vi "Source Live Profile.vi"(9 "Source Profile File":path, 10 "Simulate/Run":T1=enum."Run VI") -> (0 "error IO":errorcluster, 1 "Source Profile Out":path)   [LabVIEW 2021]
uses:
  Anemometry/Anemometry Sub Vis/Controls/User_Specific_mode.ctl
  Anemometry/Anemometry Sub Vis/Globals/Trav_pos_global.vi
  Anemometry/Anemometry Sub Vis/Globals/Meas_global.vi
panel:
  out "Initial Trace Voltage":dbl
  out "Initial Source Strength":dbl
  out "Control Trace Gas":bool
  out "Source Value":dbl format="%.2f"
  out "Time (s)":dbl[](array[numeric])
  out "XY Graph":cluster{dbl[], dbl[]}(graph)
  out "Source State":dbl[](array[numeric])
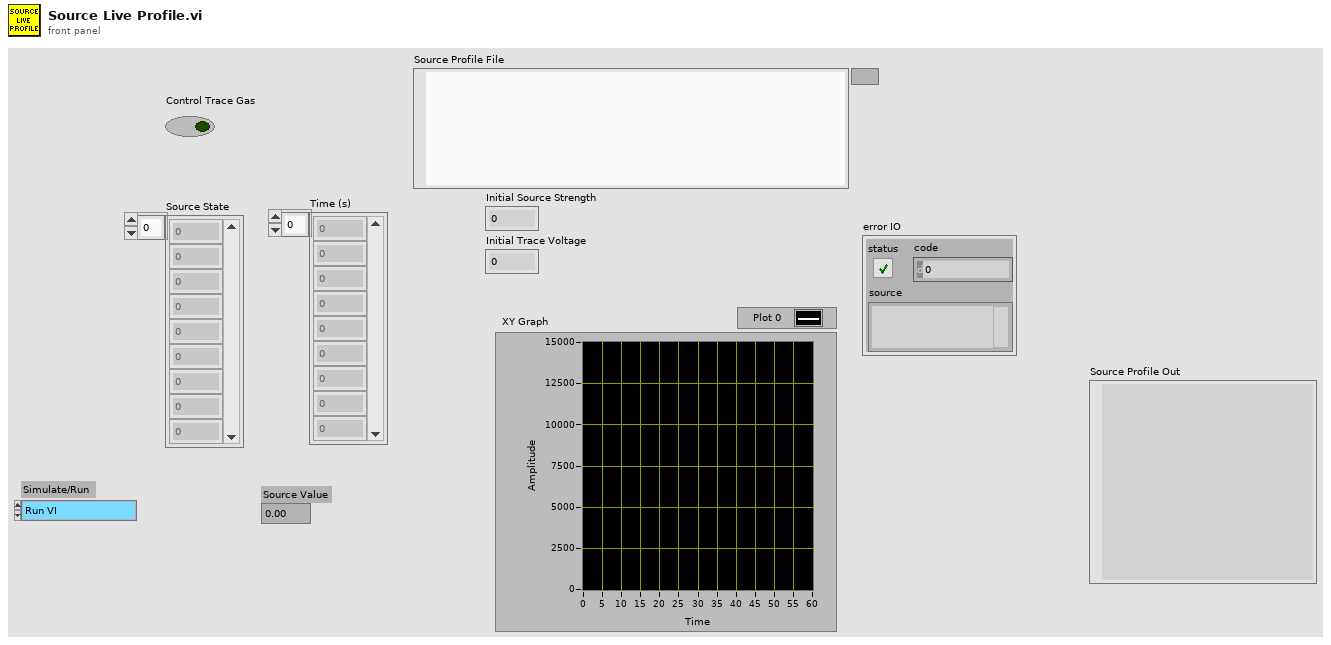
[diagram p1: front panel]
types:
  T1 = typedef "User_Specific_mode.ctl" = enum16{"Check VI only", "Run VI"}
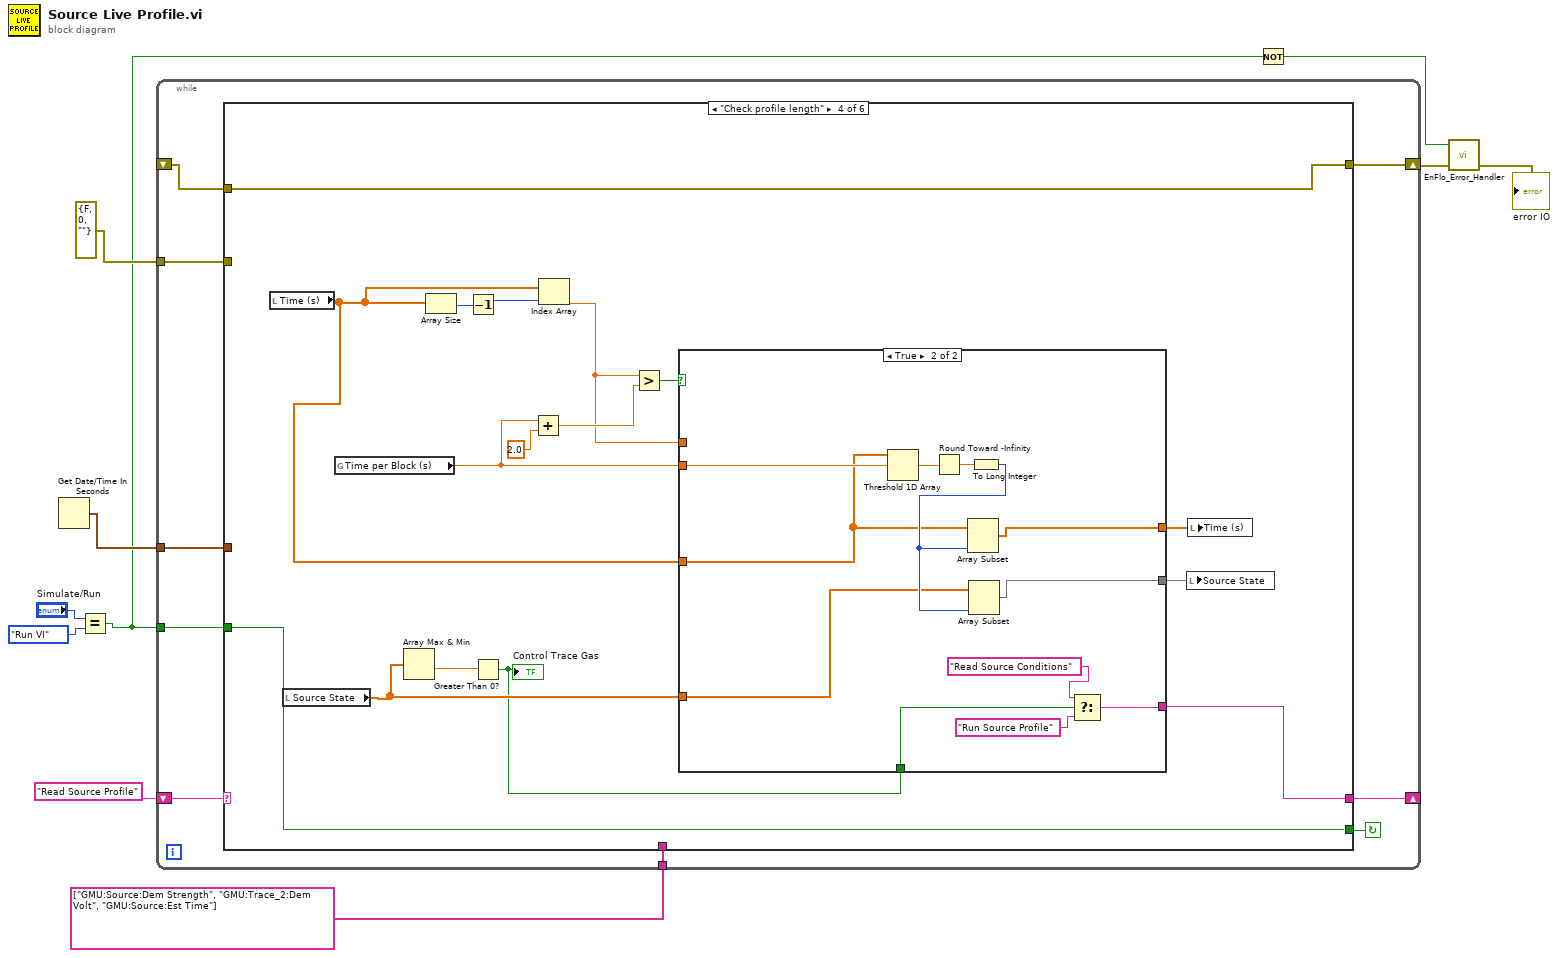
[diagram p0: block diagram]
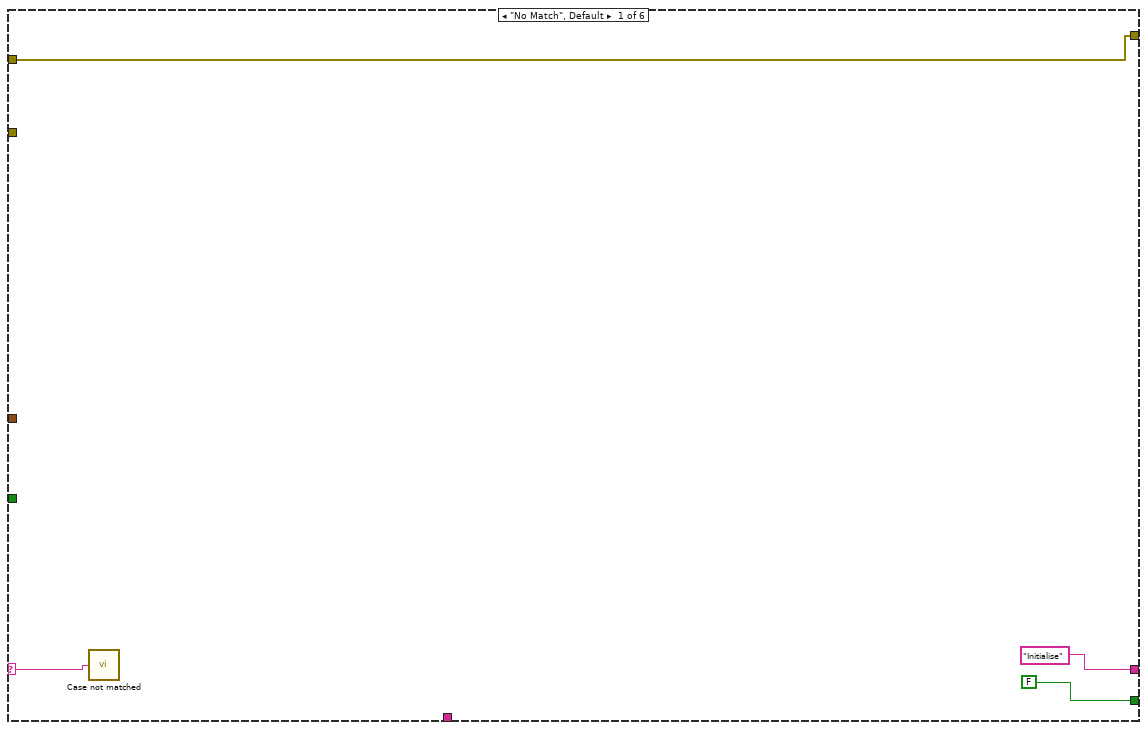
[diagram p2: hidden frame]
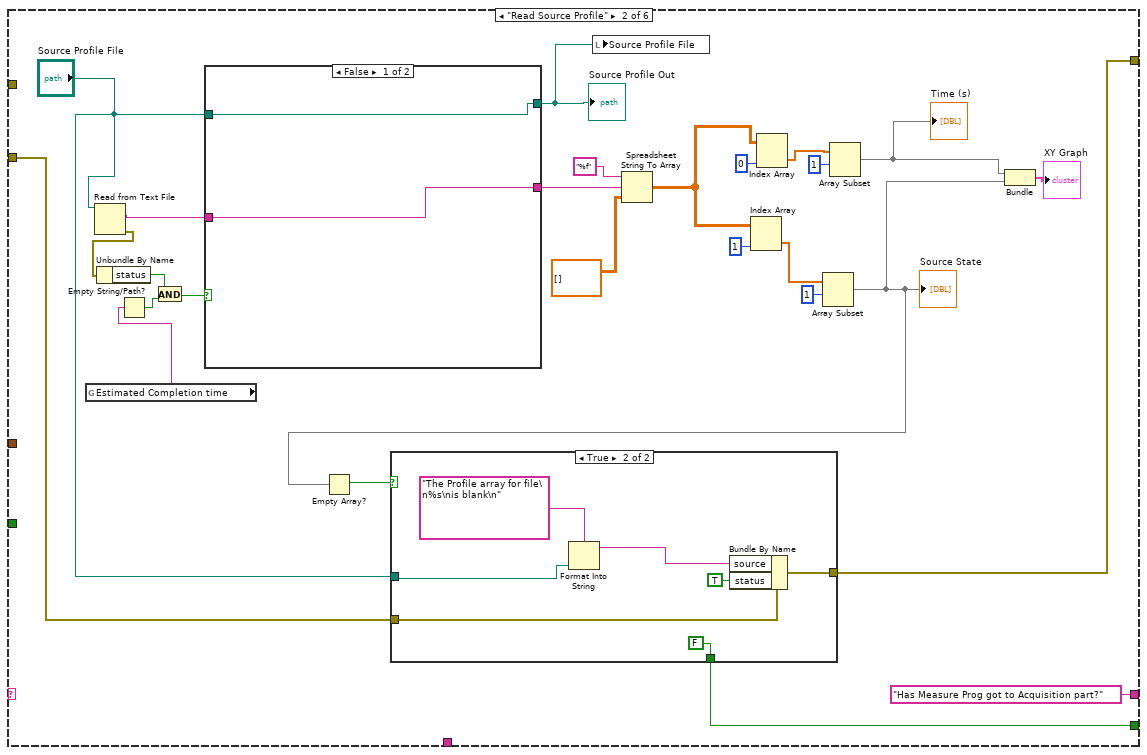
[diagram p3: hidden frame]
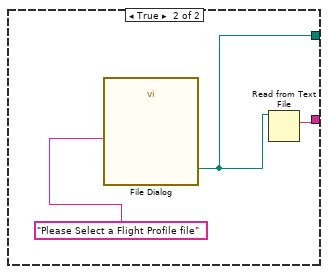
[diagram p4: hidden frame]
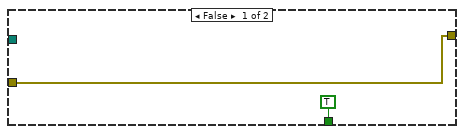
[diagram p5: hidden frame]
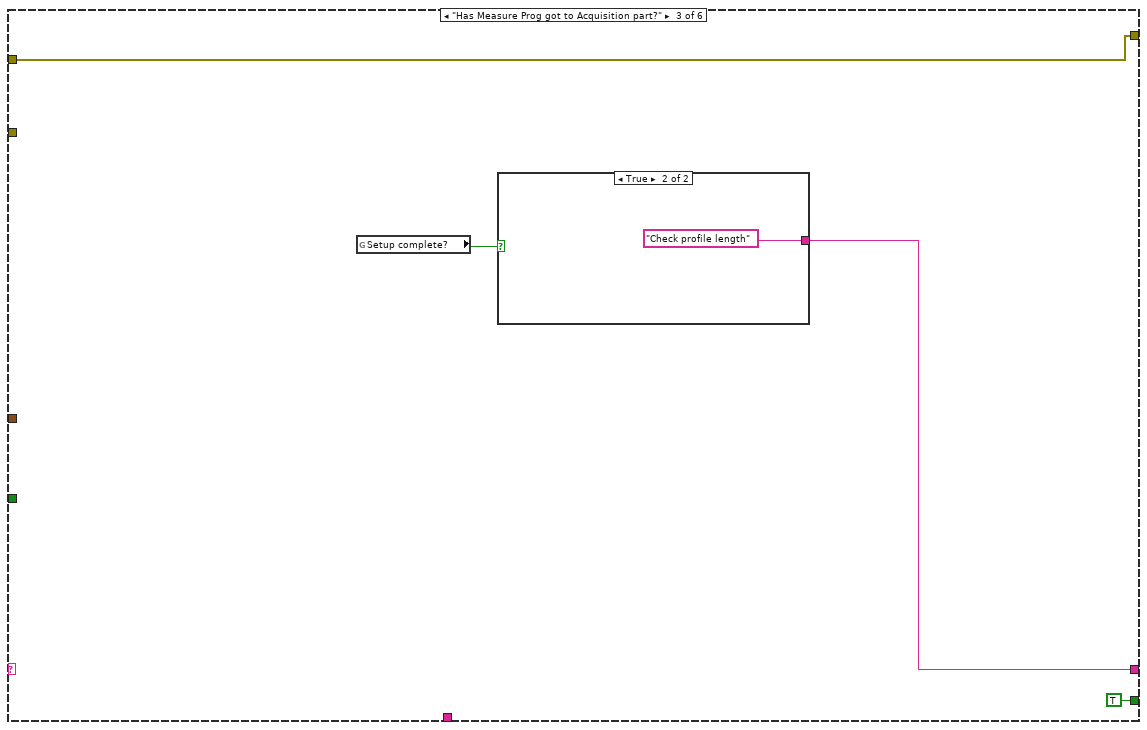
[diagram p6: hidden frame]
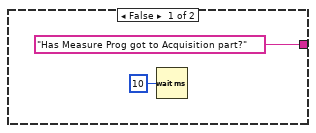
[diagram p7: hidden frame]
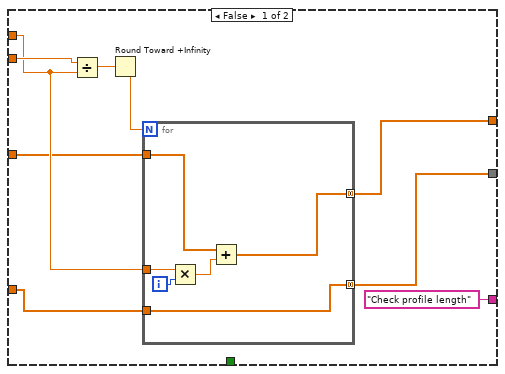
[diagram p8: hidden frame]
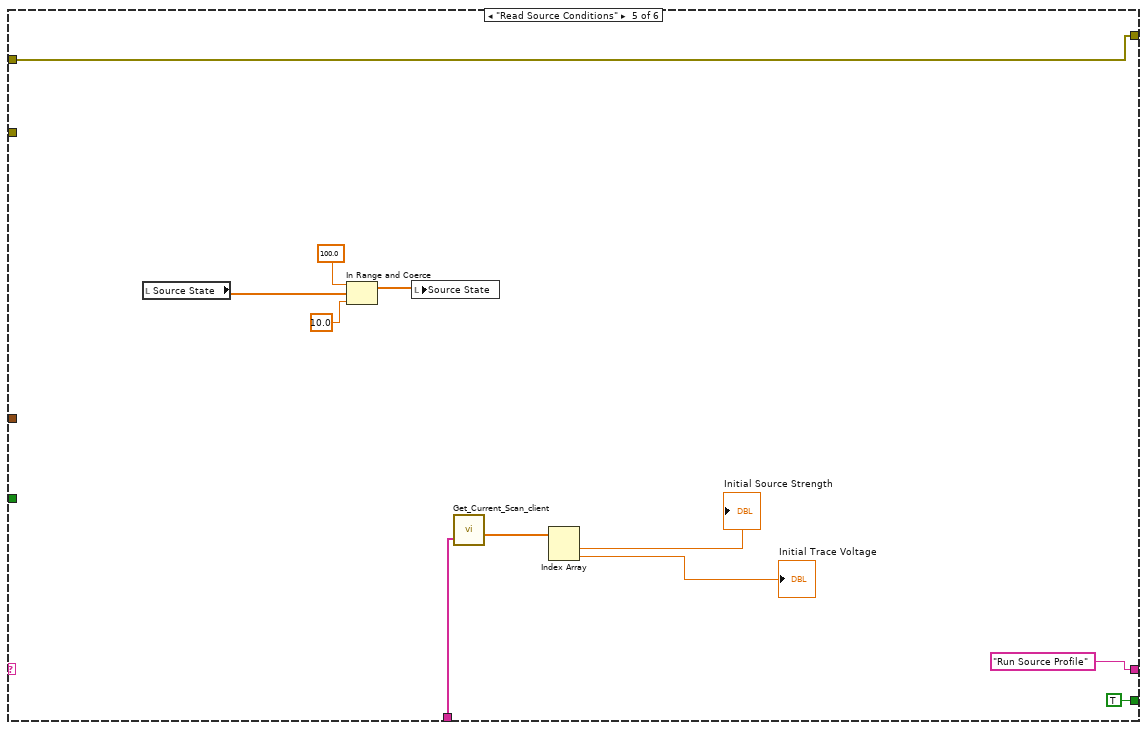
[diagram p9: hidden frame]
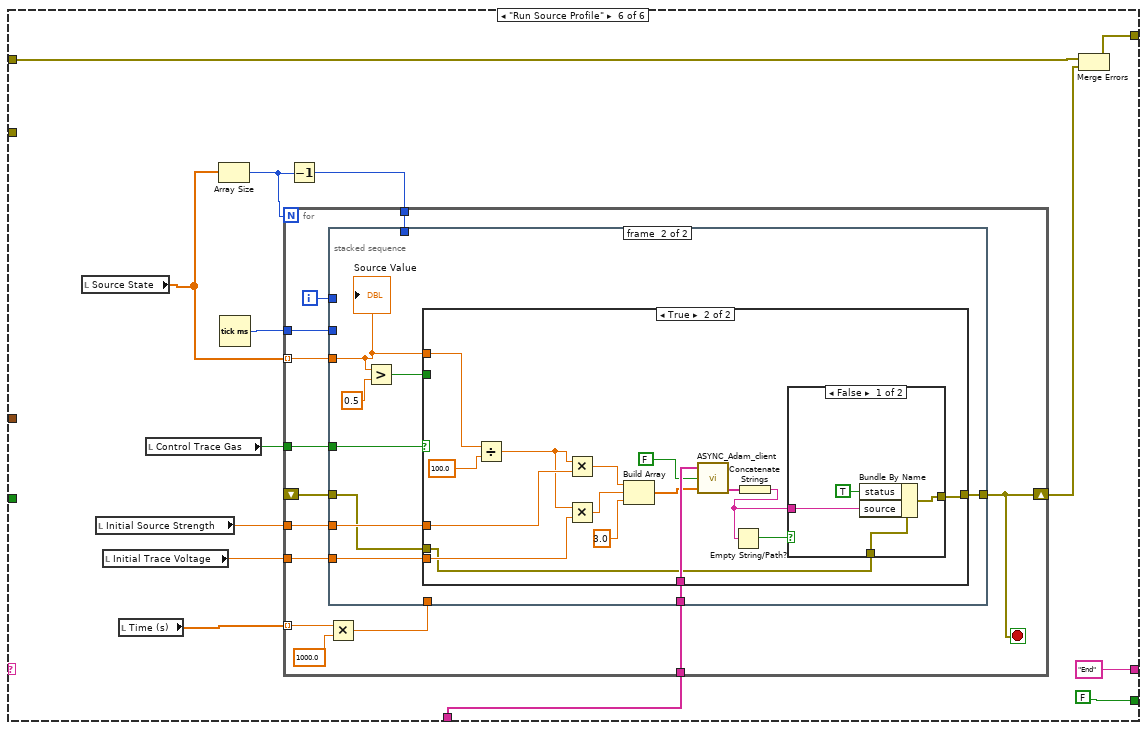
[diagram p10: hidden frame]
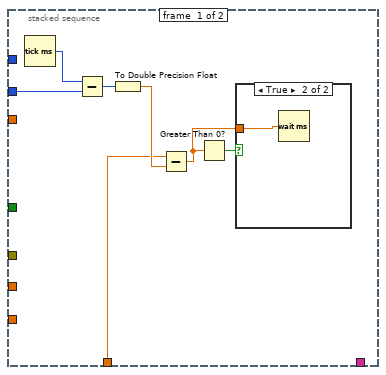
[diagram p11: hidden frame]
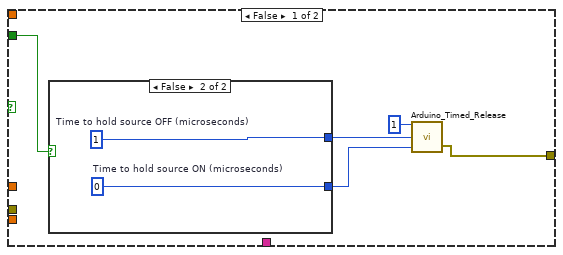
[diagram p13: hidden frame]
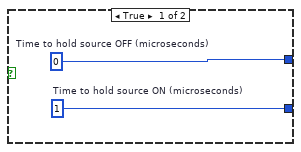
[diagram p14: hidden frame]
diagram:
  n1 = Get Date/Time In Seconds() -> (seconds since 1Jan1904=w8:timestamp)
  n2 = Equal?(x="Simulate/Run", y=User_Specific_mode."Run VI" ("Simulate/Run")) -> (x = y?=w3:bool)
  n3 = while {
    shift-left: "Read Source Profile" -> [w16]
    shift-right: [w17] -> _
    tunnel: w8 -> [w15]
    tunnel: errorcluster {"status"=FALSE, "code"=0, "source"=""} ("error in (no error)") -> [w14]
    shift-right: [w13] -> w6
    shift-left: _ -> [w12]
    tunnel: w3 -> [w11]
    tunnel: string[] ["GMU:Source:Dem Strength", "GMU:Trace_2:Dem Volt", "GMU:Source:Est Time"] -> [w10]
    stop <- w18 continue-if-true
    n4 = case shown="\"Check profile length\"" w16 {
      selector: w16 -> [w20 _ _ _ _ _]
      tunnel: [FALSE w36 TRUE w83 TRUE FALSE] -> w18
      tunnel: ["Initialise" "Has Measure Prog got to Acquisition part?" w66 w70 "Run Source Profile" "End"] -> w17
      tunnel: w15 -> [_ _ _ _ _ _]
      tunnel: w14 -> [_ w33 _ _ _ _]
      tunnel: [w19 w32 w64 w80 w118 w129] -> w13
      tunnel: w12 -> [w19 _ w64 w80 w118 w130]
      tunnel: w11 -> [_ _ _ w83 _ _]
      tunnel: w10 -> [_ _ _ _ w117 w125]
      frame "No Match", Default {
        n5 = call "Case not matched.vi"("Case Name not Matched"=w20) -> ()
      }
      frame "Read Source Profile" {
        n6 = global read "Trav_pos_global.vi" "Estimated Completion time"() -> (w28:string)
        n7 = Read from Text File(file (use dialog)="Source Profile File") -> (text=w25:string, error out=w31:errorcluster)  [unwired: 3 in, 2 out]
        n8 = Unbundle By Name(w31) -> ("status"=w30:bool)
        n9 = Empty String/Path?(string/path=w28) -> (empty?=w29:bool)
        n10 = And(x=w30, y=w29) -> (x .and. y?=w27:bool)
        n11 = case shown="False" w27 {
          tunnel: [w50 w52] -> w26
          tunnel: w25 -> [w50 _]
          tunnel: [w49 w51] -> w23
          tunnel: "Source Profile File" -> [w49 _]
          frame False {
          }
          frame True {
            n12 = call "File Dialog"("prompt"="Please Select a Flight Profile file") -> ("selected path"=w51:path)  [unwired: 11 in, 3 out]
            n13 = Read from Text File(file (use dialog)=w51) -> (text=w52:string)  [unwired: 3 in, 3 out]
          }
        }
        "Source Profile Out" <- w23
        n14 = local write "Source Profile File"(w23) -> ()
        n15 = Spreadsheet String To Array(format string="%f", spreadsheet string=w26, array type (2D Dbl)=dbl[][] []) -> (array=w47:dbl[][])  [unwired: 1 in]
        n16 = Index Array(array=w47, index (col)=1 ("disabled index (col)")) -> (element=w46:dbl[])  [unwired: 1 in]
        n17 = Index Array(array=w47, index (col)=0 ("disabled index (col)")) -> (element=w48:dbl[])  [unwired: 1 in]
        n18 = Array Subset(array=w46, index=1) -> (w38:dbl[])  [unwired: 1 in]
        "Source State" <- w38
        n19 = Empty Array?(array=w38) -> (empty?=w37:bool)
        n20 = case shown="True" w37 {
          tunnel: [TRUE FALSE] -> w36
          tunnel: "Source Profile File" -> [_ w61]
          tunnel: w33 -> [w54 w59]
          tunnel: [w54 w56] -> w32
          frame False {
          }
          frame True {
            n21 = Format Into String(format string="The Profile array for file\n%s\nis blank\n", w61) -> (resulting string=w57:string)  [unwired: 2 in, 1 out]
            n22 = Bundle By Name(cluster=w59, "source"=w57, "status"=TRUE) -> (w56:errorcluster)
          }
        }
        n23 = Array Subset(array=w48, index=1) -> (w34:dbl[])  [unwired: 1 in]
        "Time (s)" <- w34
        n24 = Bundle(w34, w38) -> (→"XY Graph":cluster{dbl[], dbl[]})  [unwired: 1 in]
      }
      frame "Has Measure Prog got to Acquisition part?" {
        n25 = global read "Meas_global.vi" "Setup complete?"() -> (w63:bool)
        n26 = case shown="True" w63 {
          tunnel: ["Has Measure Prog got to Acquisition part?" "Check profile length"] -> w66
          frame False {
            n27 = Wait (ms)(milliseconds to wait=u32 10) -> ()  [unwired: 1 out]
          }
          frame True {
          }
        }
      }
      frame "Check profile length" {
        n28 = local read "Time (s)"() -> (w72:dbl[])
        n29 = local read "Source State"() -> (w81:dbl[])
        n30 = global read "Meas_global.vi" "Time per Block (s)"() -> (w79:dbl)
        n31 = Array Max & Min(array=w81) -> (min value=w82:dbl)  [unwired: 3 out]
        n32 = Array Size(array=w72) -> (size(s)=w85:i32)
        n33 = Decrement(x=w85) -> (x-1=w84:i32)
        n34 = Greater Than 0?(x=w82) -> (x > 0?=w71:bool)
        "Control Trace Gas" <- w71
        n35 = Add(x=w79, y=2.0) -> (x+y=w76:dbl)
        n36 = Index Array(array=w72, index=w84) -> (element=w75:dbl)
        n37 = Greater?(x=w75, y=w76) -> (0:w77:bool)
        n38 = case shown="True" w77 {
          tunnel: w79 -> [w94 w110]
          tunnel: w75 -> [w92 _]
          tunnel: w81 -> [w88 w108]
          tunnel: [w90 w107] -> w74
          tunnel: [w89 w106] -> w73
          tunnel: w72 -> [w91 w105]
          tunnel: w71 -> [_ w102]
          tunnel: ["Check profile length" ("t") w101] -> w70
          frame False {
            n39 = Divide(x=w94, y=w92) -> (x/y=w93:dbl)
            n40 = Round Toward +Infinity(x=w93) -> (ceil(x): smallest int >= x=w87:dbl)
            n41 = for {
              N: w87 -> [_]
              tunnel: w92 -> [w99]
              tunnel: w91 -> [w97]
              tunnel: [w96] -> w90 mode=concatenating
              tunnel: [w95] -> w89 mode=concatenating
              tunnel: w88 -> [w95]
              i -> [w100]
              n42 = Multiply(x=w99, y=w100) -> (x*y=w98:dbl)
              n43 = Add(x=w97, y=w98) -> (x+y=w96:dbl[])
            }
          }
          frame True {
            n44 = Threshold 1D Array(2:w110, 3:w105) -> (0:w112:dbl)  [unwired: 1 in]
            n45 = Round Toward -Infinity(1:w112) -> (0:w111:dbl)
            n46 = To Long Integer(number=w111) -> (32bit integer=w109:i32)
            n47 = Array Subset(array=w105, length=w109) -> (w107:dbl[])  [unwired: 1 in]
            n48 = Array Subset(array=w108, length=w109) -> (w106:dbl[])  [unwired: 1 in]
            n49 = Select(t="Read Source Conditions", s=w102, f="Run Source Profile") -> (s? t:f=w101:string)
          }
        }
        n50 = local write "Source State"(w73) -> ()
        n51 = local write "Time (s)"(w74) -> ()
      }
      frame "Read Source Conditions" {
        n52 = local read "Source State"() -> (w114:dbl[])
        n53 = In Range and Coerce(upper limit=100.0, x=w114, lower limit=10.0) -> (coerced(x)=w113:dbl[])  [unwired: 1 out]
        n54 = local write "Source State"(w113) -> ()
        n55 = call "Get_Current_Scan_client.vi"("multipleChannels"=w117) -> ("Numerical Values"=w123:dbl[])  [unwired: 1 in, 3 out]
        n56 = Index Array(array=w123) -> (element #1=→"Initial Source Strength":dbl, element #2=→"Initial Trace Voltage":dbl)  [unwired: 2 in]
      }
      frame "Run Source Profile" {
        n57 = local read "Source State"() -> (w124:dbl[])
        n58 = local read "Initial Source Strength"() -> (w127:dbl)
        n59 = local read "Initial Trace Voltage"() -> (w126:dbl)
        n60 = local read "Time (s)"() -> (w134:dbl[])
        n61 = local read "Control Trace Gas"() -> (w128:bool)
        n62 = Array Size(array=w124) -> (size(s)=w133:i32)
        n63 = Tick Count (ms)() -> (millisecond timer value=w135:u32)
        n64 = Decrement(x=w133) -> (x-1=w132:i32)
        n65 = for {
          N: w133 -> [_]
          tunnel: w135 -> [w150]
          tunnel: w134 -> [w149] mode=indexing
          tunnel: w124 -> [w146] mode=indexing
          tunnel: w132 -> [w145]
          shift-right: [w143] -> w131
          shift-left: _ -> [w142]
          tunnel: w128 -> [w141]
          tunnel: w127 -> [w140]
          tunnel: w126 -> [w139]
          tunnel: w125 -> [w138]
          i -> [w144]
          stop <- w143 stop-if-true
          n66 = Multiply(x=w149, y=1000.0) -> (x*y=w147:dbl)
          n67 = stacked-sequence {
            tunnel: w150 -> [w156 _]
            tunnel: w147 -> [w151 _]
            tunnel: w146 -> [_ w163]
            tunnel: w145 -> [_ _]
            tunnel: w144 -> [_ _]
            tunnel: [_ w165] -> w143
            tunnel: w142 -> [_ w159]
            tunnel: w141 -> [_ w164]
            tunnel: w140 -> [_ w162]
            tunnel: w139 -> [_ w161]
            tunnel: w138 -> [_ w160]
            frame #0 {
              n68 = Tick Count (ms)() -> (millisecond timer value=w157:u32)
              n69 = Subtract(x=w157, y=w156) -> (x-y=w155:u32)
              n70 = To Double Precision Float(number=w155) -> (double precision float=w154:dbl)
              n71 = Subtract(x=w151, y=w154) -> (x-y=w152:dbl)
              n72 = Greater Than 0?(x=w152) -> (x > 0?=w153:bool)
              n73 = case shown="True" w153 {
                tunnel: w152 -> [_ w158]
                frame False {
                }
                frame True {
                  n74 = Wait (ms)(milliseconds to wait=w158) -> ()  [unwired: 1 out]
                }
              }
            }
            frame #1 {
              n75 = Greater?(x=w163, y=0.5) -> (0:w166:bool)
              n76 = case shown="True" w164 {
                tunnel: w166 -> [w169 _]
                tunnel: [w168 w180] -> w165
                tunnel: w163 -> [_ w192]
                tunnel: w162 -> [_ w190]
                tunnel: w161 -> [_ w188]
                tunnel: w160 -> [_ w187]
                tunnel: w159 -> [_ w179]
                frame False {
                  n77 = case shown="False" w169 {
                    tunnel: [w174 w176] -> w171
                    tunnel: [w173 w175] -> w172
                    frame True {
                      w173 = u32 0  # Time to hold source OFF (microseconds)
                      w174 = u32 1  # Time to hold source ON (microseconds)
                    }
                    frame False {
                      w175 = u32 1  # Time to hold source OFF (microseconds)
                      w176 = u32 0  # Time to hold source ON (microseconds)
                    }
                  }
                  n78 = call "Arduino_Timed_Release.vi"("Time to hold source ON (microseconds)"=w171, "Time to hold source OFF (microseconds)"=w172, "Number of cycles"=u16 1) -> ("error out"=w168:errorcluster)  [unwired: 1 out]
                }
                frame True {
                  n79 = Divide(x=w192, y=100.0) -> (x/y=w189:dbl)
                  n80 = Multiply(x=w189, y=w190) -> (x*y=w185:dbl)
                  n81 = Multiply(x=w189, y=w188) -> (x*y=w184:dbl)
                  n82 = Build Array(w185, w184, 3.0 ("element")) -> (w183:dbl[])
                  n83 = call "ASYNC_Adam_client.vi"("Values"=w183, "Check Value is in the scan table?"=FALSE, "Channel Names"=w187) -> ("Scan Comments"=w182:string[])  [unwired: 1 out]
                  n84 = Concatenate Strings(w182) -> (w178:string)
                  n85 = Empty String/Path?(string/path=w178) -> (empty?=w181:bool)
                  n86 = case shown="False" w181 {
                    tunnel: [w195 w197] -> w180
                    tunnel: w179 -> [w196 w197]
                    tunnel: w178 -> [w194 _]
                    frame False {
                      n87 = Bundle By Name(cluster=w196, "status"=TRUE, "source"=w194) -> (w195:errorcluster)
                    }
                    frame True {
                    }
                  }
                }
              }
              "Source Value" <- w163
            }
          }
        }
        n88 = Merge Errors(w130, w131) -> (w129:errorcluster)
      }
    }
  }
  "error IO" <- w6
  n89 = Not(x=w3) -> (.not. x?=w2:bool)
  n90 = call "EnFlo_Error_Handler.vi"("error in (no error)"=w6, "Dialog Box (F)"=w2) -> ()  [unwired: 2 in, 2 out]
